vi "Get Error Description.vi"(11 "error source":string) -> (3 "error description":string)   [LabVIEW 2021, in "MeasurementClient Editor.lvlib"]
uses:
  MeasurementClient Editor.lvlib
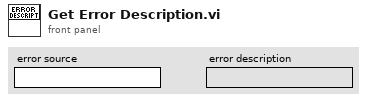
[diagram p1: front panel]
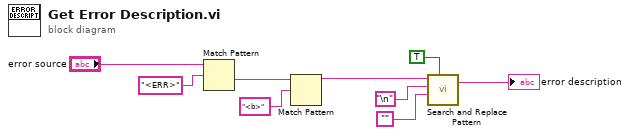
[diagram p0: block diagram]
diagram:
  n1 = Match Pattern(string="error source", regular expression="<ERR>") -> (after substring=w6:string)  [unwired: 1 in, 3 out]
  n2 = Match Pattern(string=w6, regular expression="<b>") -> (before substring=w5:string)  [unwired: 1 in, 3 out]
  n3 = call <vilib>:"Search and Replace Pattern.vi"("string"=w5, "regular expression (\"\")"="\n", "replace string (\"\")"="", "replace all? (F)"=TRUE) -> ("result string"=→"error description":string)  [unwired: 1 in, 1 out]
